vi "Set Telemetry Services.vi"(9 "RemoteDataService":refnum<class "RemoteDataService.lvclass">, 10 "ChannelService":refnum<class "ChannelService.lvclass">, 11 "VolatusAPI in":refnum<class "VolatusAPI.lvclass">) -> (3 "VolatusAPI out":refnum<class "VolatusAPI.lvclass">)   [LabVIEW 2020, in "Volatus.lvlib" / "VolatusAPI.lvclass"]
uses:
  VolatusAPI.lvclass
  lv-vecto/Vecto/ChannelService/ChannelService.lvclass
  lv-vecto/Vecto/RemoteDataService/RemoteDataService.lvclass
  VolatusAPI.lvclass/VolatusAPI.ctl
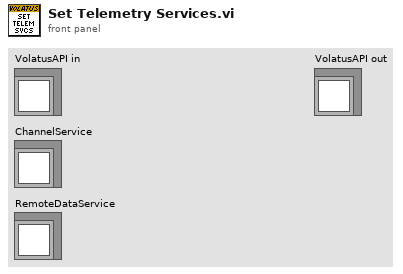
[diagram p1: front panel]
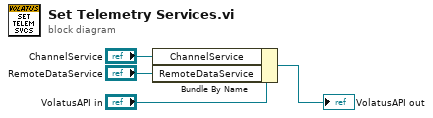
[diagram p0: block diagram]
diagram:
  n1 = Bundle By Name(cluster="VolatusAPI in", "ChannelService"="ChannelService", "RemoteDataService"="RemoteDataService") -> (→"VolatusAPI out":refnum<class "VolatusAPI.lvclass">)
